vi "HiCCE_Display_v1_4.vi"() -> ()   [LabVIEW 2019]
uses:
  <vilib>/Analysis/3filter.llb/Filter Passband Type.ctl
  <vilib>/Analysis/4window.llb/windowTd.ctl
  <vilib>/Analysis/3filter.llb/Butterworth Filter (DBL).vi
  <vilib>/Analysis/0measdsp.llb/Scaled Time Domain Window (DBL).vi
  <vilib>/Analysis/NI_AALPro.lvlib
  <vilib>/Analysis/NI_AALBase.lvlib
panel:
  out "element 2":u8
  out "element":u8
  out "size(s)":i32
  out "decimal integer string":string[](array[string])
  out "Array":dbl[](array[numeric])
  out "Oscilloscope":u32[](array[numeric])
  out "STATUS":u32
  out "DEC_STATUS 2":u8[](array[numeric])
  out "DEC_STATUS":u8[](array[numeric])
  in  "TF display enable":bool
  in  "Numeric":i32
  in  "Load Button":bool
  in  "save\n Button":bool
  out "sampals/transfer":i32
  in  "order 2":i32=2
  in  "low cutoff freq: fl 2":dbl=0.12500000000000006 format="%0.4f"
  in  "high cutoff freq: fh 2":dbl=0.45000000000000007 format="%0.2f"
  in  "filter type 2":T1
  in  "no. seg(x512)":i32
  in  "Ch No.":i32
  in  "window 2":T2 items=["Rectangle"=0, "Hanning"=1, "Hamming"=2, "Blackman-Harris"=3, "Exact Blackman"=4, "Blackman"=5, "Flat Top"=6, "4 Term B-Harris "=7, "7 Term B-Harris"=8, "Low Sidelobe"=9, "Blackman Nuttall"=11, "Triangle"=30, "Bartlett-Hanning"=31, "Bohman"=32, "Parzen"=33, "Welch"=34, "Kaiser"=60, "Dolph-Chebyshev"=61, "Gaussian"=62]
  in  "Window length":i32(slide)=57 scale=10.0..1024.0
  in  "high cutoff freq: fh":dbl=0.45000000000000007 format="%0.2f"
  in  "order":i32=2
  in  "low cutoff freq: fl":dbl=0.12500000000000006 format="%0.4f"
  out "Display time filterd (ms)":dbl
  in  "filter type":T1
  out "Waveform Chart 3":dbl[](graph)
  in  "Channel No.":dbl
  out "Plot No. 2":i32
  out "Display Time (ms)":dbl
  in  "sampling rate (kHz)":dbl
  in  "Windowed":bool
  in  "stop":bool
  out "Waveform Chart 2":u32[](graph)
  out "*(type *) &x":u32[](array[numeric]) format="%x"
  out "Waveform Chart":u32[][](graph)
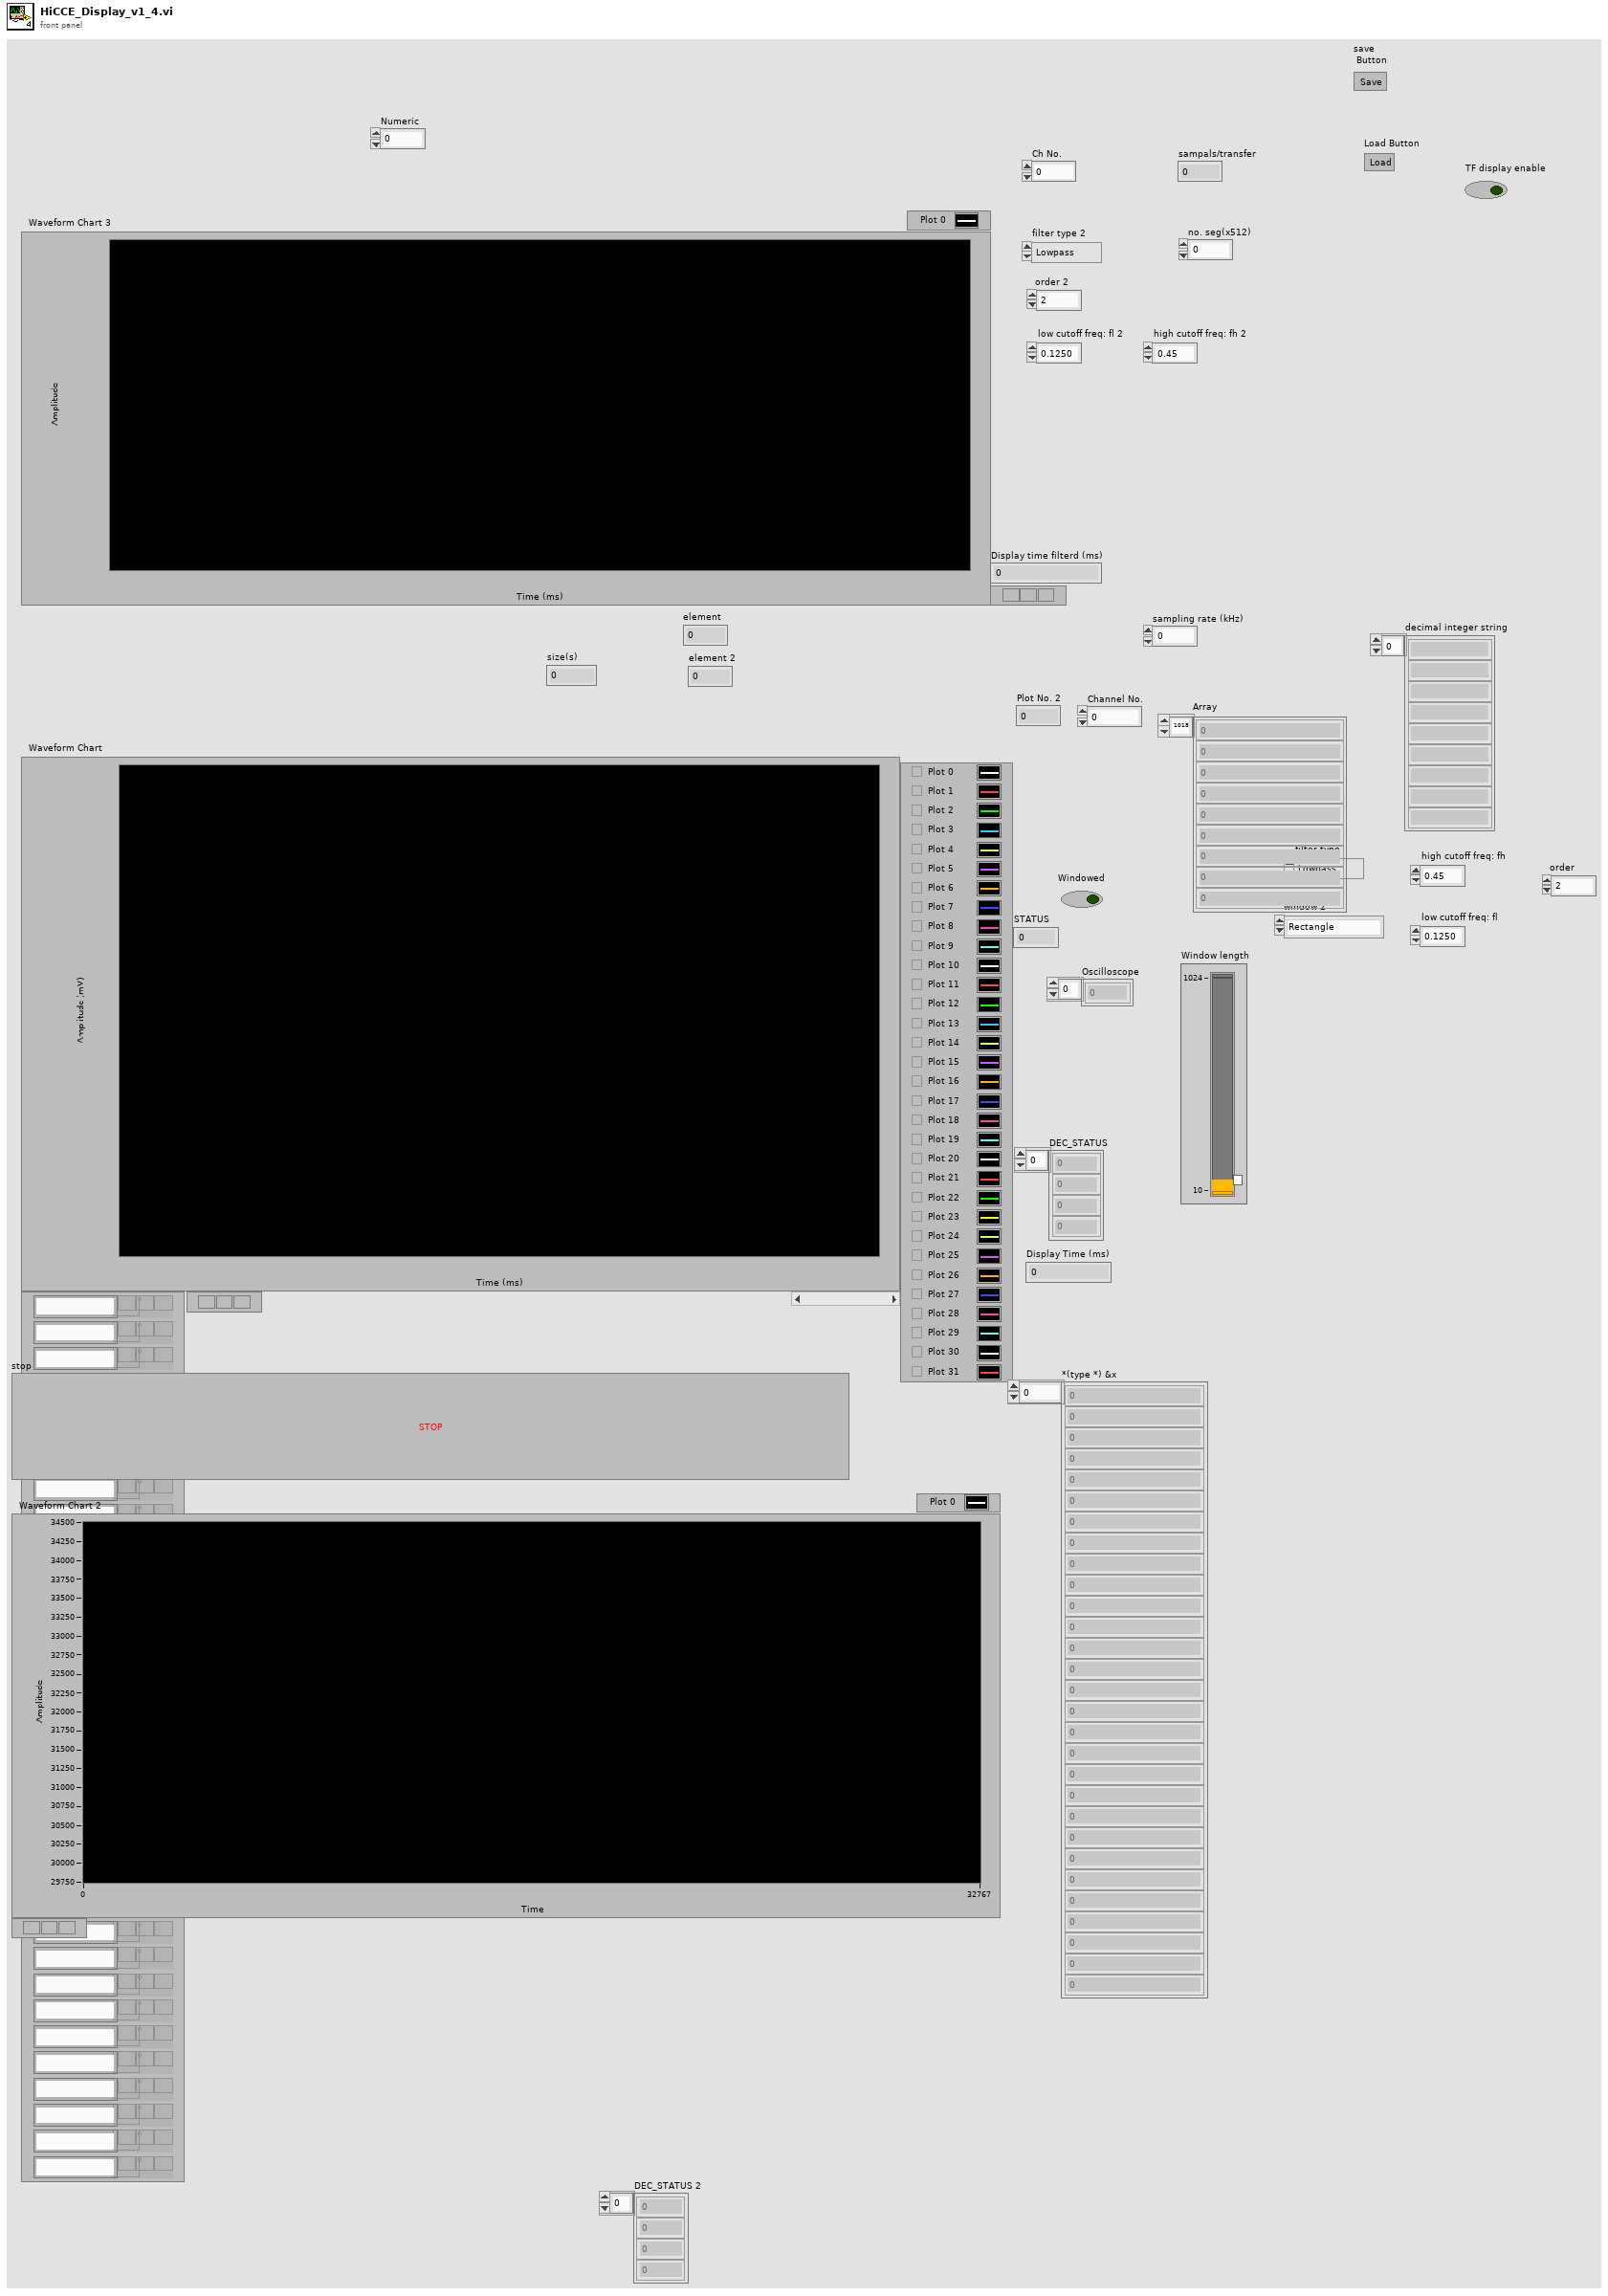
[diagram p1: front panel]
types:
  T1 = typedef "NI_AALBase.lvlib/Filter Passband Type.ctl" = enum32{"Lowpass", "Highpass", "Bandpass", "Bandstop"}
  T2 = typedef "NI_AALPro.lvlib/windowTd.ctl" = u32
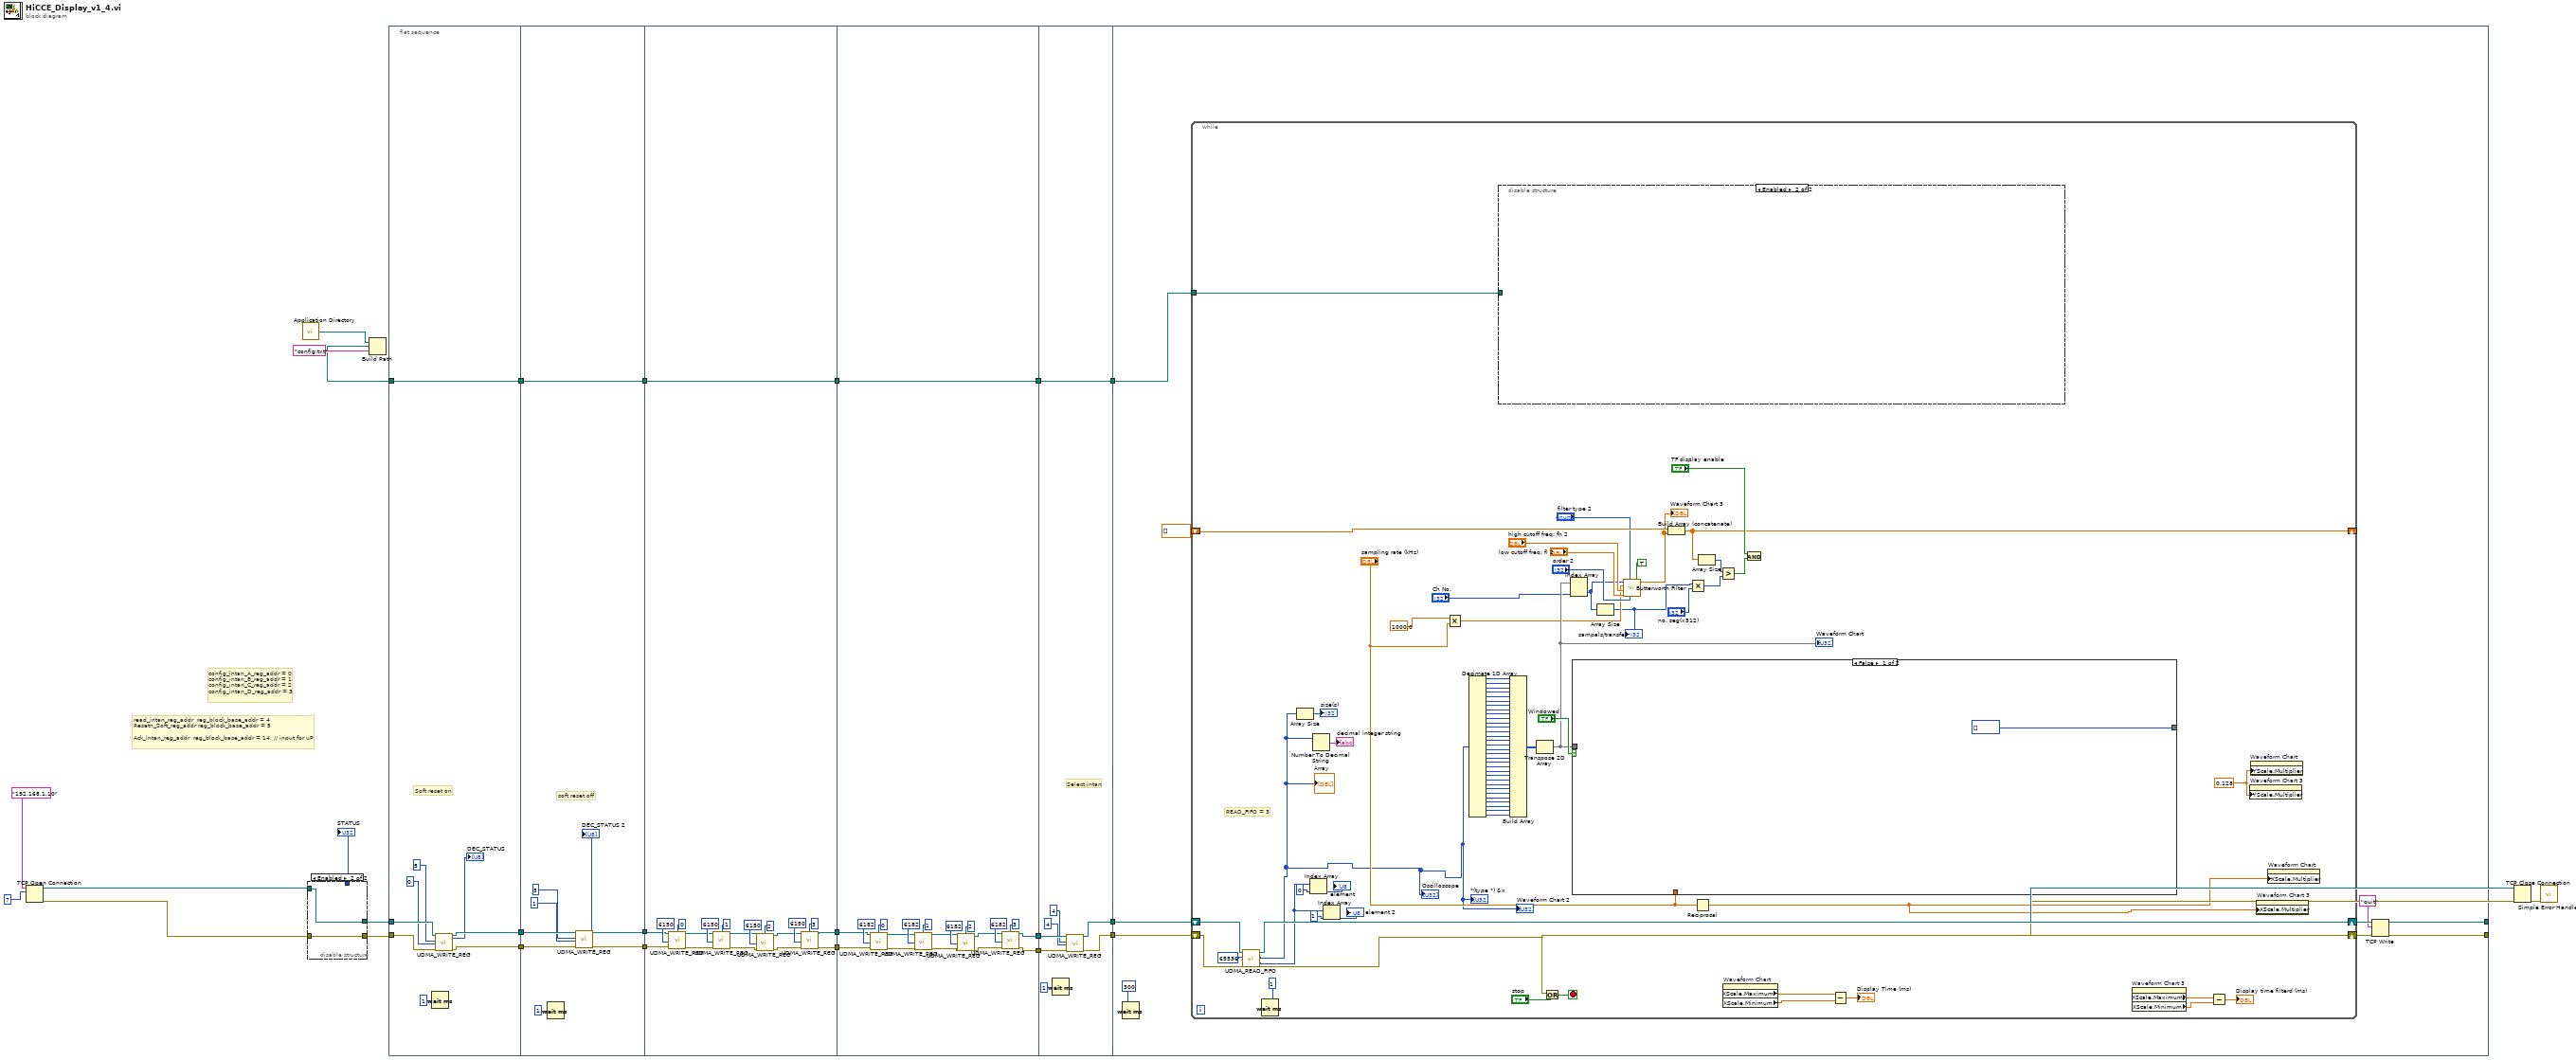
[diagram p0: block diagram]
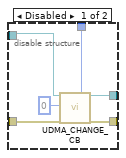
[diagram p2: hidden frame]
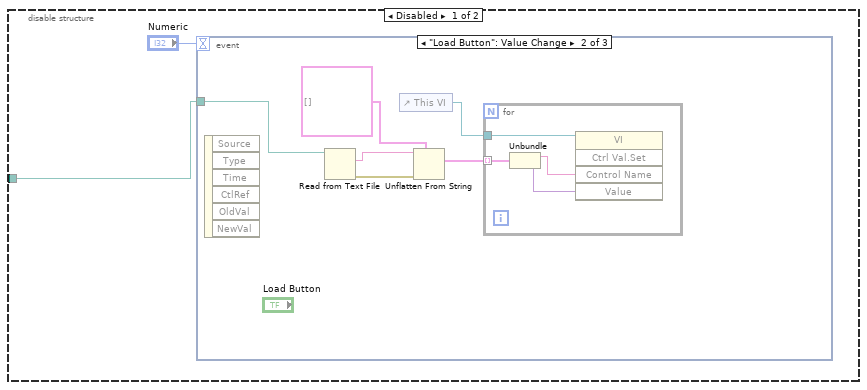
[diagram p3: hidden frame]
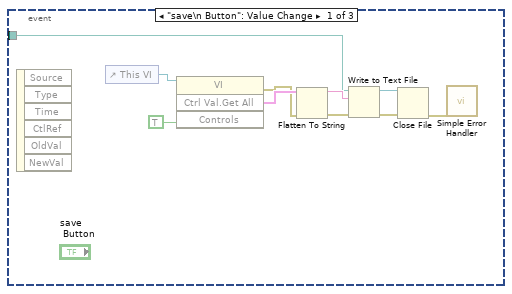
[diagram p4: hidden frame]
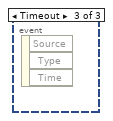
[diagram p5: hidden frame]
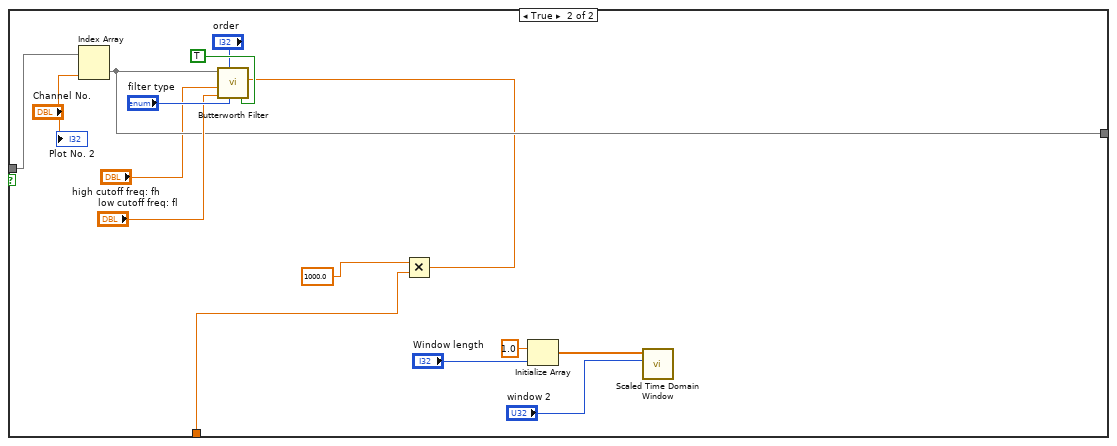
[diagram p6: hidden frame]
diagram:
  # "read_intan_reg_addr\t\treg_block_base_addr = 4\nResetn_Soft_reg_addr\treg_block_base_addr = 5\n\nAck_intan_reg_addr\t\treg_block_base_addr = 14\t\t// input for uP"
  # "config_intan_A_reg_addr = 0\nconfig_intan_B_reg_addr = 1\nconfig_intan_C_reg_addr = 2\nconfig_intan_D_reg_addr = 3"
  n1 = TCP Open Connection(address="192.168.1.10", remote port or service name=u16 7) -> (connection ID=w7:refnum<k5>, error out=w6:errorcluster)  [unwired: 3 in]
  n2 = call <vilib>:"Application Directory.vi"() -> ("Application Directory"=w23:path)
  n3 = disable-structure shown="Enabled" {
    disable-tunnel: w7 -> [w34 w36]
    disable-tunnel: w6 -> [w33 w35]
    disable-tunnel: [w31 w36] -> w5
    disable-tunnel: [w30 w35] -> w4
    disable-tunnel: [w29 _] -> w3
    frame Disabled {
      n4 = call "UDMA_CHANGE_CB.vi"("TCP Network Connection in"=w34, "CB_ID"=u32 0, "error in (no error)"=w33) -> ("TCP Network Connection out"=w31:refnum<k5>, "STATUS"=w29:u32, "error out"=w30:errorcluster)  [unwired: 14 in]
    }
    frame Enabled {
    }
  }
  "STATUS" <- w3
  n5 = Build Path(base path=w23, name or relative path="config.txt") -> (appended path=w21:path)
  n6 = flat-sequence {
    tunnel: w21 -> [w45]
    tunnel: [w45] -> w20
    tunnel: w5 -> [w43]
    tunnel: w4 -> [w42]
    tunnel: [w39] -> w15
    tunnel: [w38] -> w14
    tunnel: w20 -> [w54]
    tunnel: [w54] -> w19
    tunnel: w15 -> [w52]
    tunnel: w14 -> [w51]
    tunnel: [w47] -> w13
    tunnel: [w46] -> w12
    tunnel: [w73] -> w11
    tunnel: w19 -> [w73]
    tunnel: w13 -> [w61]
    tunnel: w12 -> [w60]
    tunnel: [w56] -> w9
    tunnel: [w55] -> w8
    tunnel: w11 -> [w92]
    tunnel: [w92] -> w10
    tunnel: w9 -> [w77]
    tunnel: w8 -> [w76]
    tunnel: [w75] -> w2
    tunnel: [w74] -> w1
    tunnel: [w94] -> w18
    tunnel: [w93] -> w17
    tunnel: w10 -> [w100]
    tunnel: [w100] -> w16
    tunnel: w2 -> [w98]
    tunnel: w1 -> [w97]
    tunnel: [w104] -> w26
    tunnel: [w103] -> w25
    tunnel: w18 -> [w110]
    tunnel: w17 -> [w109]
    tunnel: w16 -> [w101]
    frame #0 {
      # "Soft reset on"
      n7 = Wait (ms)(milliseconds to wait=u32 1) -> ()  [unwired: 1 out]
      n8 = call "UDMA_WRITE_REG.vi"("TCP Network Connection in"=w43, "REG"=u32 5, "DATA"=u32 0, "error in (no error)"=w42) -> ("TCP Network Connection out"=w39:refnum<k5>, "DEC_STATUS"=→"DEC_STATUS":u8[], "error out"=w38:errorcluster)  [unwired: 13 in]
    }
    frame #1 {
      # "soft reset off"
      n9 = Wait (ms)(milliseconds to wait=u32 1) -> ()  [unwired: 1 out]
      n10 = call "UDMA_WRITE_REG.vi"("TCP Network Connection in"=w52, "REG"=u32 5, "DATA"=u32 1, "error in (no error)"=w51) -> ("TCP Network Connection out"=w47:refnum<k5>, "DEC_STATUS"=→"DEC_STATUS 2":u8[], "error out"=w46:errorcluster)  [unwired: 13 in]
    }
    frame #2 {
      n11 = call "UDMA_WRITE_REG.vi"("TCP Network Connection in"=w61, "REG"=u32 0, "DATA"=u32 6150, "error in (no error)"=w60) -> ("TCP Network Connection out"=w64:refnum<k5>, "error out"=w59:errorcluster)  [unwired: 13 in, 1 out]
      n12 = call "UDMA_WRITE_REG.vi"("TCP Network Connection in"=w64, "REG"=u32 1, "DATA"=u32 6150, "error in (no error)"=w59) -> ("TCP Network Connection out"=w63:refnum<k5>, "error out"=w58:errorcluster)  [unwired: 13 in, 1 out]
      n13 = call "UDMA_WRITE_REG.vi"("TCP Network Connection in"=w63, "REG"=u32 2, "DATA"=u32 6150, "error in (no error)"=w58) -> ("TCP Network Connection out"=w62:refnum<k5>, "error out"=w57:errorcluster)  [unwired: 13 in, 1 out]
      n14 = call "UDMA_WRITE_REG.vi"("TCP Network Connection in"=w62, "REG"=u32 3, "DATA"=u32 6150, "error in (no error)"=w57) -> ("TCP Network Connection out"=w56:refnum<k5>, "error out"=w55:errorcluster)  [unwired: 13 in, 1 out]
    }
    frame #3 {
      n15 = call "UDMA_WRITE_REG.vi"("TCP Network Connection in"=w77, "REG"=u32 0, "DATA"=u32 6182, "error in (no error)"=w76) -> ("TCP Network Connection out"=w83:refnum<k5>, "error out"=w80:errorcluster)  [unwired: 13 in, 1 out]
      n16 = call "UDMA_WRITE_REG.vi"("TCP Network Connection in"=w83, "REG"=u32 1, "DATA"=u32 6182, "error in (no error)"=w80) -> ("TCP Network Connection out"=w82:refnum<k5>, "error out"=w79:errorcluster)  [unwired: 13 in, 1 out]
      n17 = call "UDMA_WRITE_REG.vi"("TCP Network Connection in"=w82, "REG"=u32 2, "DATA"=u32 6182, "error in (no error)"=w79) -> ("TCP Network Connection out"=w81:refnum<k5>, "error out"=w78:errorcluster)  [unwired: 13 in, 1 out]
      n18 = call "UDMA_WRITE_REG.vi"("TCP Network Connection in"=w81, "REG"=u32 3, "DATA"=u32 6182, "error in (no error)"=w78) -> ("TCP Network Connection out"=w75:refnum<k5>, "error out"=w74:errorcluster)  [unwired: 13 in, 1 out]
    }
    frame #4 {
      # "Select intan"
      n19 = Wait (ms)(milliseconds to wait=u32 1) -> ()  [unwired: 1 out]
      n20 = call "UDMA_WRITE_REG.vi"("TCP Network Connection in"=w98, "REG"=u32 4, "DATA"=u32 4, "error in (no error)"=w97) -> ("TCP Network Connection out"=w94:refnum<k5>, "error out"=w93:errorcluster)  [unwired: 13 in, 1 out]
    }
    frame #5 {
      n21 = Wait (ms)(milliseconds to wait=u32 300) -> ()  [unwired: 1 out]
      n22 = while {
        shift-right: [w114] -> w106
        shift-left: w110 -> [w116]
        shift-right: [w111] -> w105
        shift-left: w109 -> [w115]
        shift-right: [w125] -> _
        shift-left: dbl[] [] -> [w146]
        tunnel: w101 -> [w128]
        stop <- w156 stop-if-true
        w147 = 0.128 ("Y Scale.Offset and Multiplier:Multiplier")
        # "READ_FIFO = 3"
        n23 = call "UDMA_READ_FIFO.vi"("TCP Network Connection in"=w116, "N"=u32 65536, "error in (no error)"=w115) -> ("TCP Network Connection out"=w114:refnum<k5>, "Oscilloscope"=w113:u32[], "Status"=w112:u8[], "error out"=w111:errorcluster)  [unwired: 13 in]
        "*(type *) &x" <- w113
        "Waveform Chart 2" <- w113
        "Oscilloscope" <- w113
        "Array" <- w113
        n24 = Wait (ms)(milliseconds to wait=u32 1) -> ()  [unwired: 1 out]
        n25 = Array Size(array=w113) -> (size(s)=→"size(s)":i32)
        n26 = Index Array(array=w112, index=0) -> (element=→"element":u8)
        n27 = Number To Decimal String(number=w113) -> (decimal integer string=→"decimal integer string":string[])  [unwired: 1 in]
        n28 = Index Array(array=w112, index=1) -> (element=→"element 2":u8)
        n29 = Multiply(x=1000.0, y="sampling rate (kHz)") -> (x*y=w134:dbl)
        n30 = Decimate 1D Array(w113) -> (w189:u32[], w188:u32[], w187:u32[], w186:u32[], w185:u32[], w184:u32[], w183:u32[], w182:u32[], w181:u32[], w180:u32[], w179:u32[], w178:u32[], w177:u32[], w176:u32[], w175:u32[], w174:u32[], w173:u32[], w172:u32[], w171:u32[], w170:u32[], w169:u32[], w168:u32[], w167:u32[], w166:u32[], w165:u32[], w164:u32[], w163:u32[], w162:u32[], w161:u32[], w160:u32[], w159:u32[], w158:u32[])
        n31 = disable-structure shown="Enabled" {
          disable-tunnel: w128 -> [w191 _]
          frame Disabled {
            n32 = event shown="[1] \"Load Button\": Value Change" {
              selector: _ -> [_ _ _]
              dyn-events: _ -> [_ _ _]
              timeout: "Numeric" -> [_ _ _]
              tunnel: w191 -> [w195 w207 _]
              event "save\n Button": Value Change {
                n33 = event-data() -> ()  [unwired: 1 in, 6 out]
                n34 = control-ref of="This VI"() -> (w201:refnum<vi>)
                n35 = invoke class="VI" method="Ctrl Val.Get All"(reference=w201, "Controls"=TRUE) -> (error out=w198:errorcluster, "Get All Control Values Variant"=w199:cluster{"Name":string, "Variant Data":variant}[])  [unwired: 2 in, 2 out]
                n36 = Flatten To String(anything=w199, error in (no error)=w198) -> (data string=w197:string, error out=w196:errorcluster)  [unwired: 2 in, 1 out]
                n37 = Write to Text File(file (use dialog)=w195, text=w197, error in=w196) -> (refnum out=w194:refnum<file>, error out=w193:errorcluster)  [unwired: 1 in, 1 out]
                n38 = Close File(refnum=w194, error in=w193) -> (error out=w192:errorcluster)  [unwired: 1 out]
                n39 = call <vilib>:"Simple Error Handler.vi"("error in (no error)"=w192) -> ()  [unwired: 4 in, 5 out]
              }
              event "Load Button": Value Change {
                n40 = event-data() -> ()  [unwired: 1 in, 6 out]
                n41 = Read from Text File(file (use dialog)=w207) -> (text=w206:string, error out=w205:errorcluster)  [unwired: 3 in, 2 out]
                n42 = control-ref of="This VI"() -> (w202:refnum<vi>)
                n43 = Unflatten From String(type=cluster{string, variant}[] [], binary string=w206, error in (no error)=w205) -> (value=w203:cluster{string, variant}[])  [unwired: 2 in, 2 out]
                n44 = for {
                  tunnel: w203 -> [w211] mode=indexing
                  tunnel: w202 -> [w210]
                  n45 = Unbundle(w211) -> (w209:string, w208:variant)
                  n46 = invoke class="VI" method="Ctrl Val.Set"(reference=w210, "Control Name"=w209, "Value"=w208) -> ()  [unwired: 2 in, 5 out]
                }
              }
              event Timeout {
                n47 = event-data() -> ()  [unwired: 1 in, 3 out]
              }
            }
          }
          frame Enabled {
          }
        }
        n48 = Build Array(w189, w188, w187, w186, w185, w184, w183, w182, w181, w180, w179, w178, w177, w176, w175, w174, w173, w172, w171, w170, w169, w168, w167, w166, w165, w164, w163, w162, w161, w160, w159, w158) -> (w157:u32[][])
        n49 = Transpose 2D Array(2D array=w157) -> (transposed array=w145:u32[][])
        "Waveform Chart" <- w145
        n50 = Or(x=w111, y="stop") -> (x .or. y?=w156:bool)
        n51 = Index Array(array=w145, index (col)="Ch No.") -> (element=w133:u32[])  [unwired: 1 in]
        n52 = case shown="False" "Windowed" {
          tunnel: w145 -> [_ w227]
          tunnel: "sampling rate (kHz)" -> [_ w224]
          tunnel: [u32[] [] w221] -> _
          frame False {
          }
          frame True {
            n53 = Index Array(array=w227, index (col)="Channel No.") -> (element=w221:u32[])  [unwired: 1 in]
            n54 = Multiply(x=1000.0, y=w224) -> (x*y=w215:dbl)
            n55 = call-poly <vilib>:"Butterworth Filter.vi"("init/cont (init:F)"=TRUE, "order"="order", "filter type"="filter type", "low cutoff freq: fl"="low cutoff freq: fl", "high cutoff freq: fh"="high cutoff freq: fh", "sampling freq: fs"=w215, "X"=w221) -> ()  [unwired: 1 in, 2 out]
            n56 = Initialize Array(1.0 ("element"), "Window length") -> (w218:dbl[])
            n57 = call-poly <vilib>:"Scaled Time Domain Window.vi"("window"="window 2", "X"=w218) -> ()  [unwired: 1 in, 9 out]
            "Plot No. 2" <- "Channel No."
          }
        }
        n58 = Array Size(array=w133) -> (size(s)=w132:i32)
        "sampals/transfer" <- w132
        n59 = call-poly <vilib>:"Butterworth Filter.vi"("init/cont (init:F)"=TRUE, "order"="order 2", "filter type"="filter type 2", "low cutoff freq: fl"="low cutoff freq: fl 2", "high cutoff freq: fh"="high cutoff freq: fh 2", "sampling freq: fs"=w134, "X"=w133) -> ("Filtered X"=w135:dbl[])  [unwired: 1 in, 1 out]
        "Waveform Chart 3" <- w135
        n60 = Build Array (concatenate)(w146, w135) -> (w125:dbl[])
        n61 = Multiply(x=w132, y="no. seg(x512)") -> (x*y=w130:i32)
        n62 = Reciprocal(x="sampling rate (kHz)") -> (1/x=w129:dbl)
        n63 = Array Size(array=w125) -> (size(s)=w143:i32)
        n64 = Greater?(x=w143, y=w130) -> (0:w127:bool)
        n65 = property on="Waveform Chart" class="WFChart (strict)"() -> ("XScale.Maximum"=w153:dbl, "XScale.Minimum"=w152:dbl)  [unwired: 2 in, 2 out]
        n66 = And(x="TF display enable", y=w127) -> ()  [unwired: 1 out]
        n67 = Subtract(x=w153, y=w152) -> (x-y=→"Display Time (ms)":dbl)
        n68 = property on="Waveform Chart 3" class="WFChart (strict)"() -> ("XScale.Maximum"=w150:dbl, "XScale.Minimum"=w149:dbl)  [unwired: 2 in, 2 out]
        n69 = Subtract(x=w150, y=w149) -> (x-y=→"Display time filterd (ms)":dbl)
        n70 = property on="Waveform Chart 3" class="WFChart (strict)"("YScale.Multiplier"=w147) -> ()  [unwired: 2 in, 2 out]
        n71 = property on="Waveform Chart" class="WFChart (strict)"("YScale.Multiplier"=w147) -> ()  [unwired: 2 in, 2 out]
        n72 = property on="Waveform Chart 3" class="WFChart (strict)"("XScale.Multiplier"=w129) -> ()  [unwired: 2 in, 2 out]
        n73 = property on="Waveform Chart" class="WFChart (strict)"("XScale.Multiplier"=w129) -> ()  [unwired: 2 in, 2 out]
      }
      n74 = TCP Write(connection ID=w106, data in="quit", error in (no error)=w105) -> (connection ID out=w104:refnum<k5>, error out=w103:errorcluster)  [unwired: 1 in, 1 out]
    }
  }
  n75 = TCP Close Connection(connection ID=w26, error in (no error)=w25) -> (error out=w24:errorcluster)  [unwired: 1 in, 1 out]
  n76 = call <vilib>:"Simple Error Handler.vi"("error in (no error)"=w24) -> ()  [unwired: 4 in, 5 out]
